vi "Run Test.vi"(8 "error in (no error)":errorcluster, 11 "Test Template in":refnum<class "Program I2C Driver.lvclass">) -> (0 "error out":errorcluster, 1 "Positions":i32[](array[numeric]), 2 "Tests Passed":bool[](array[boolean]), 3 "Test Template out":refnum<class "Program I2C Driver.lvclass">, 5 "Fail Codes":string[](array[string]))   [LabVIEW 2015, in "Program I2C Driver.lvclass"]
uses:
  Program I2C Driver.lvclass
  CBTF Applications/Utility Applications/Main/Stand-Alone I2C Programmer/Application/Application/Class/typedefs/Instrument Selector -- Enum.ctl
  Classes/Programmer/I2C Programmer/Class/I2C Programmer.lvclass
  Classes/Instruments/I2C Device/NI-8451/NI-8451.lvclass
  Classes/Application/Class/Application.lvclass
  Test Class/Test Class.lvclass
  CBTF Applications/Utility Applications/Main/Stand-Alone I2C Programmer/Application/Application/Class/I2C Programmer.lvclass
  <vilib>/Cree, Inc/Cree Test Framework/Classes/Base Objects/Base Class/Base Class/Base Class.lvclass
  Classes/Programmer/Programmer/Class/Programmer.lvclass
  Classes/Test Recipe/Class/Test Recipe.lvclass
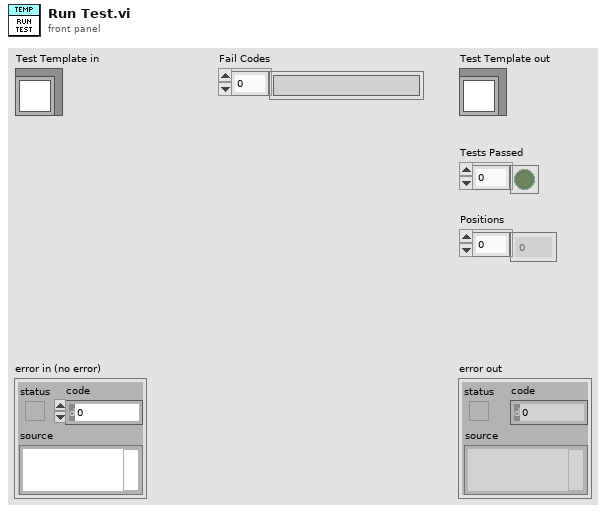
[diagram p1: front panel]
types:
  T1 = typedef "I2C Programmer App.lvlib/I2C Programmer.lvclass/Instrument Selector -- Enum.ctl" = enum16{"I2C Device", ""}
  T2 = typedef "Application.lvlib/App Properties.lvclass/Class Properties -- Cluster.ctl" = cluster{"UUT Info":T3[], "Test Information":refnum<vi>, "Test Complete Event":refnum<user-event>, "Shop Floor System":refnum<class "Shop Floor System.lvclass">, "Gold Board":refnum<class "Golden Board.lvclass">, "Test Recipe":refnum<class "Test Recipe.lvclass">, "Instruments":refnum<class "Instrument.lvclass">[], "Mode":T4, "Test Results":T5[], "Station Config":refnum<class "Station Config.lvclass">, "Variable Engine":refnum<class "Variable Engine.lvclass">}
  T3 = typedef "Application.lvlib/App Properties.lvclass/UUT Reference -- Cluster.ctl" = cluster{"Serial Number Reference":refnum<vi>, "Status Message Reference":refnum<vi>}
  T4 = typedef "Application.lvlib/Application.lvclass/Op Mode -- Enum.ctl" = u16
  T5 = typedef "Application.lvlib/App Properties.lvclass/Test Result -- Cluster.ctl" = cluster{"Position":i32, "Pass":bool, "Fail Codes":string}
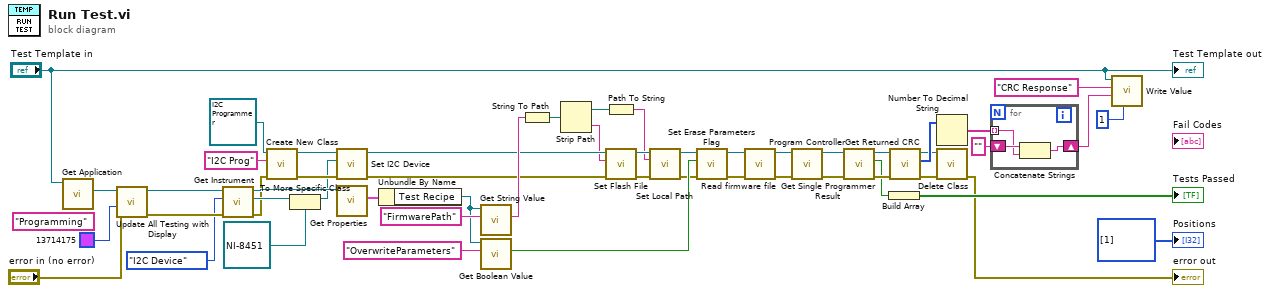
[diagram p0: block diagram]
diagram:
  (unwired) "Programming" ("Message ('')")
  n1 = call "Get Application.vi"("Test Class in"="Test Template in") -> ("Application.lvlib:Application.lvclass"=w7:refnum<class "Application.lvclass">)  [unwired: 9 in, 1 out]
  n2 = call "Update All Testing with Display.vi"("error in (no error)"="error in (no error)", "BG Color"=u32 13714175, "Application in"=w7) -> ("error out"=w19:errorcluster, "Application out"=w18:refnum<class "Application.lvclass">)  [unwired: 7 in]
  n3 = call "Get Instrument.vi"("error in (no error)"=w19, "Instrument Number"=Instrument_Selector_--_Enum."I2C Device" ("Instrument"), "Application in"=w18) -> ("error out"=w12:errorcluster, "Instrument"=w14:refnum<class "Instrument.lvclass">, "Application out"=w27:refnum<class "Application.lvclass">)  [unwired: 6 in]
  n4 = call <vilib>:"Create New Class.vi"("error in (no error)"=w12, "Name"="I2C Prog", "Base Class in"=refnum<class "I2C Programmer.lvclass"> refnum ("I2C Programmer.lvlib:I2C Programmer.lvclass")) -> ("error out"=w17:errorcluster, "Base Class out"=w13:refnum<class "I2C Programmer.lvclass">)  [unwired: 7 in]
  n5 = To More Specific Class(target class=refnum<class "NI-8451.lvclass"> refnum ("NI-8451.lvlib:NI-8451.lvclass"), reference=w14) -> (specific class reference=w16:refnum<class "NI-8451.lvclass">)  [unwired: 1 in, 1 out]
  n6 = call "Set I2C Device.vi"("error in (no error)"=w17, "I2C Device.lvlib:I2C Device.lvclass"=w16, "I2C Programmer in"=w13) -> ("error out"=w25:errorcluster, "I2C Programmer out"=w24:refnum<class "I2C Programmer.lvclass">)  [unwired: 7 in]
  n7 = call "Get Properties.vi"("Acrobat Template in"=w27) -> ("Class Properties"=w28:T2)  [unwired: 8 in, 2 out]
  n8 = Unbundle By Name(w28) -> ("Test Recipe"=w32:refnum<class "Test Recipe.lvclass">)
  n9 = call "Get String Value.vi"("Name"="FirmwarePath", "Test Recipe in"=w32) -> ("Value"=w29:string)  [unwired: 6 in, 3 out]
  n10 = call "Get Boolean Value.vi"("Name"="OverwriteParameters", "Test Recipe in"=w32) -> ("Value"=w35:bool)  [unwired: 6 in, 3 out]
  n11 = String To Path(string=w29) -> (path=w30:path)
  n12 = Strip Path(path=w30) -> (stripped path=w23:path, name=w21:string)
  n13 = Path To String(path=w23) -> (string=w20:string)
  n14 = call "Set Flash File.vi"("error in (no error)"=w25, "Flash File"=w21, "Programmer in"=w24) -> ("error out"=w26:errorcluster, "Programmer out"=w22:refnum<class "I2C Programmer.lvclass">)  [unwired: 7 in]
  n15 = call "Set Local Path.vi"("error in (no error)"=w26, "Local Path"=w20, "Programmer in"=w22) -> ("error out"=w6:errorcluster, "Programmer out"=w31:refnum<class "I2C Programmer.lvclass">)  [unwired: 7 in]
  n16 = call "Set Erase Parameters Flag.vi"("error in (no error)"=w6, "Erase Parameters"=w35, "I2C Programmer in"=w31) -> ("error out"=w38:errorcluster, "I2C Programmer out"=w37:refnum<class "I2C Programmer.lvclass">)  [unwired: 7 in]
  n17 = call-dynamic "Read firmware file.vi"("error in (no error)"=w38, "I2C Programmer in"=w37) -> ("error out"=w39:errorcluster, "I2C Programmer out"=w36:refnum<class "I2C Programmer.lvclass">)  [unwired: 8 in]
  n18 = call-dynamic "Program Controller.vi"("error in (no error)"=w39, "I2C Programmer in"=w36) -> ("error out"=w41:errorcluster, "I2C Programmer out"=w40:refnum<class "I2C Programmer.lvclass">)  [unwired: 8 in]
  n19 = call-dynamic "Get Single Programmer Result.vi"("error in (no error)"=w41, "Programmer in"=w40) -> ("error out"=w44:errorcluster, "Success"=w42:bool, "Programmer out"=w43:refnum<class "I2C Programmer.lvclass">)  [unwired: 6 in, 1 out]
  n20 = Build Array(w42) -> (→"Tests Passed":bool[])
  n21 = call "Get Returned CRC.vi"("error in (no error)"=w44, "I2C Programmer in"=w43) -> ("error out"=w45:errorcluster, "Returned CRC"=w48:u8[], "I2C Programmer out"=w46:refnum<class "I2C Programmer.lvclass">)  [unwired: 7 in]
  n22 = Number To Decimal String(number=w48) -> (decimal integer string=w49:string[])  [unwired: 1 in]
  n23 = call <vilib>:"Delete Class.vi"("error in (no error)"=w45, "Base Class in"=w46) -> ("error out"=→"error out":errorcluster)  [unwired: 8 in, 1 out]
  n24 = for {
    tunnel: w49 -> [w53] mode=indexing
    shift-right: [w54] -> w51
    shift-left: "" ("Name") -> [w55]
    n25 = Concatenate Strings(w55, w53) -> (w54:string)
  }
  n26 = call "Write Value.vi"("Position"=1, "Value"=w51, "Label"="CRC Response", "Test Class in"="Test Template in") -> ()  [unwired: 7 in, 1 out]
  "Test Template out" <- "Test Template in"
  "Positions" <- i32[] [1]
